vi "Main.vi"   [LabVIEW 2018]
doc: "Main interface to Dataflow DJ.\n\n<b>Execution System:</b> User Interface"
uses:
  Libraries/Audio Engine/Audio Engine.lvlib
  Libraries/Audio Output/Audio Output Queue Type.ctl
  Libraries/Audio Output/Audio Output.lvlib
  Libraries/Globals/Constants.vi
  Libraries/Globals/Globals.lvlib
  Libraries/User Interface/Sub Panels Cluster.ctl
  Libraries/User Interface/User Interface.lvlib
  Libraries/Config File/Config File.lvlib
  Libraries/Track Info/Track Info.lvlib
  Libraries/Track Info/Track Info FGV Enum.ctl
  Libraries/Track Info/Track Info.ctl
  Libraries/Config File/Config Cluster.ctl
  Plugins/Controllers/DAQmx/DAQmx.lvlib
  <vilib>/Analysis/NI_AALBase.lvlib
  <vilib>/Analysis/1siggen.llb/Ramp Pattern by Samples.vi
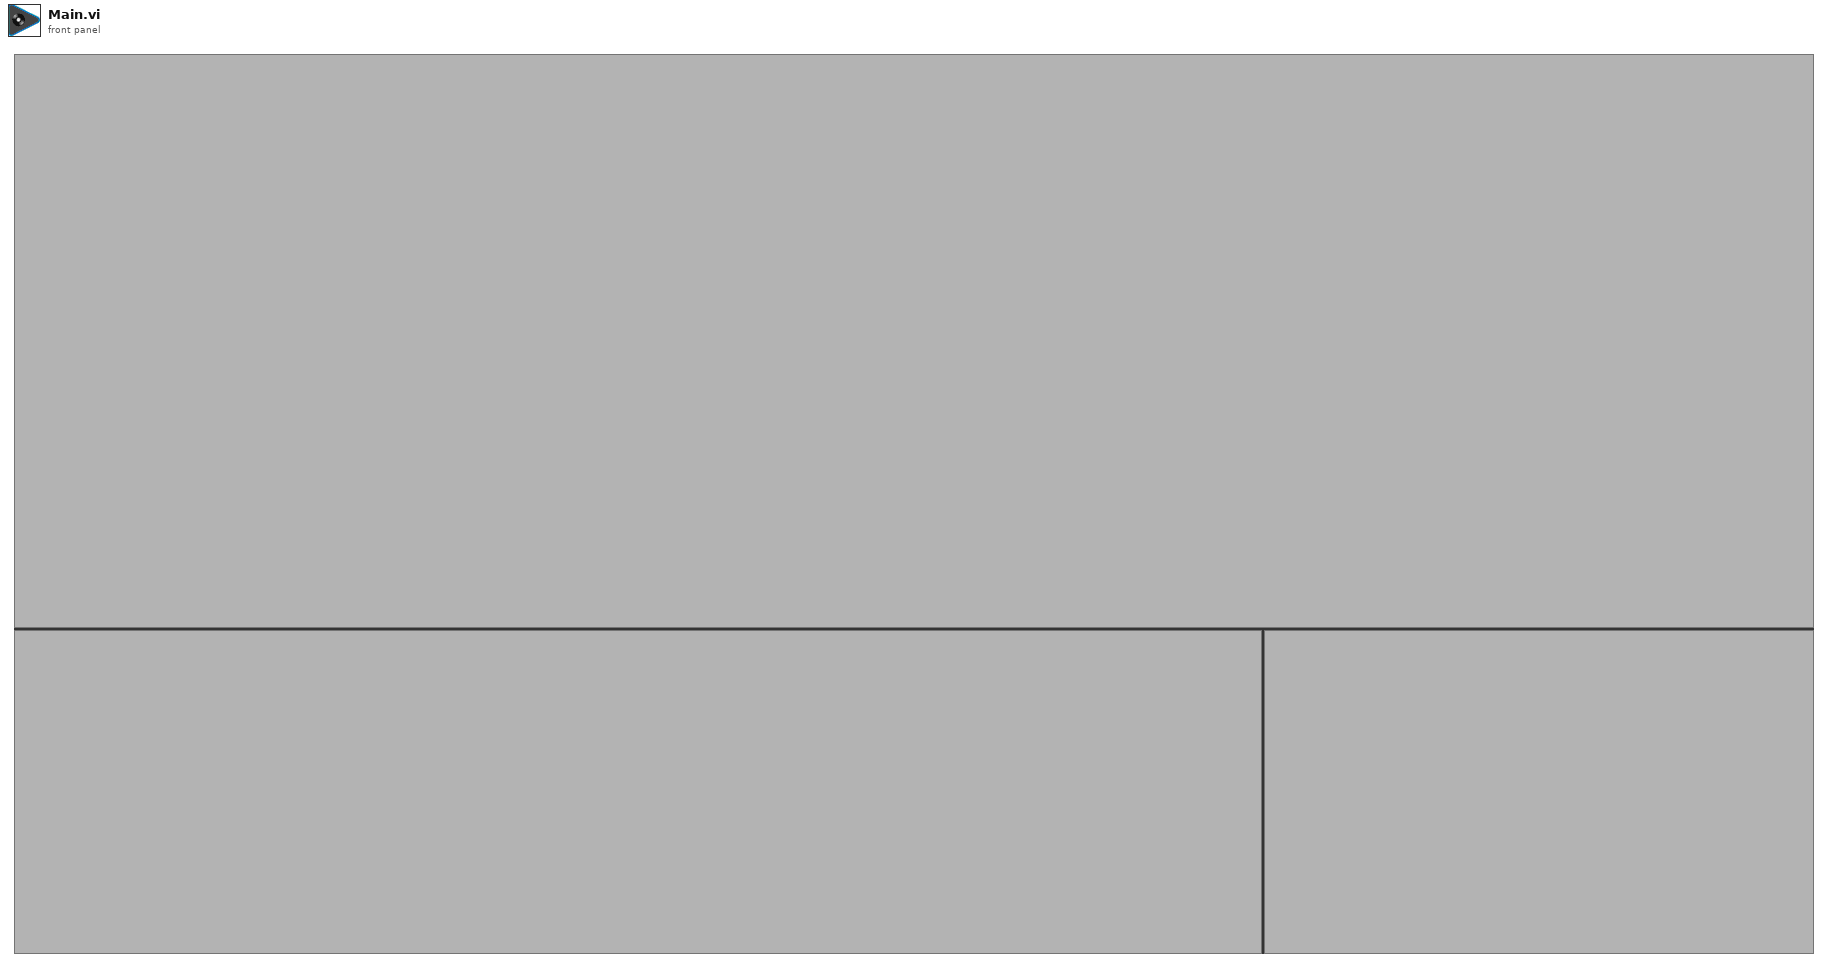
[diagram p1: front panel]
types:
  T1 = typedef "User Interface.lvlib/Sub Panels Cluster.ctl" = cluster{"DJ Interface":refnum<vi>, "File Browser":refnum<vi>, "Audio Config":refnum<vi>}
  T2 = typedef "Track Info.lvlib/Track Info FGV Enum.ctl" = enum16{"Init", "Update Track", "Update Multiple Tracks", "Get Track", "Get Multiple Tracks"}
  T3 = typedef "Audio Output.lvlib/Audio Output Queue Type.ctl" = cluster{"Master":waveform(i16)[], "Headphones":waveform(i16)[]}
  T4 = typedef "Config File.lvlib/Config Cluster.ctl" = cluster{"Track Info":T5[]}
  T5 = typedef "Track Info.lvlib/Track Info.ctl" = cluster{"Path":path, "Length (Samples)":i32, "Channels":i32, "Sample Rate (Hz)":i32, "BPM":dbl, "Cue Points (Samples)":i32[]}
  T6 = enum32{"invalid app kind", "Development System", "Run Time System", "Student Edition", "Embedded LabVIEW", "Evaluation", "Custom"}
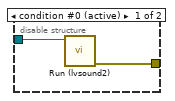
[diagram p4: hidden frame]
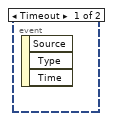
[diagram p5: hidden frame]
diagram:
  w10 = FALSE  # Shutdown
  # "Load WaveIO VIs programmatically\n\nif waveio.dll exists, then dynamically call VIs in waveio.llb\nif it doesn't exist, fall back to lvsound2.dll\n\nshould also address this issue"
  # "#TODO\nProgrammatically open reference to any VIs containing calls to DAQmx. Need to bundle those VIs with exe (block diagram included). Perform initial check for daqmx dll, and only then load VIs.\n\nUse PPLs to store code? Seem rather cumbersome to use. That said, if they're being loaded programmatically, they don't need to be linked in the project."
  # "Startup order required\nAudio Processing\n- Setup message queues for all control messages from UI and hardware\n- Begin generating output data\nAutio Output\n- Setup message queue from audio config UI panel\nUser Interface (DJ Interface)\n- Setup message queue to receive UI changes\n- Scan all UI elements and send values and limits to Audio Processing\nHardware Controller\n- Setup hardware and read current IO state\n- Send IO state to Audio Processing, which will then relay changes back to UI\n\n#TODO Use named Notifiers to wait for each component to start up"
  # "EXECUTION SYSTEMS\n\nAudio Processing.Run.vi    Standard\nAudio Output.Run.vi    Instrument I/O\nMain.vi    User Interface\nUser Interface.DJ Interface.vi    User Interface\nUser Interface.File Browser.vi    User Interface\nUser Interface.Audio Config.vi    User Interface\nHardware Control.DAQmx Run.vi    Data Acquisition\nAudio File Input.Load Async.vi    Other 1"
  # "Dataflow DJ - A live DJ mixing application written entirely in LabVIEW.\n    Copyright (C) 2019  Dataflow G\n    \n    This program is free software: you can redistribute it and/or modify\n    it under the terms of the GNU General Public License as published by\n    the Free Software Foundation, either version 3 of the License, or\n    (at your option) any later version.\n\n    This program is distributed in the hope that it will be useful,\n    but WITHOUT ANY WARRANTY; without even the implied warranty of\n    MERCHANTABILITY or FITNESS FOR A PARTICULAR PURPOSE.  See the\n    GNU General Public License for more details.\n\n    You should have received a copy of the GNU General Public License\n    along with this program.  If not, see <https://www.gnu.org/licenses/>.\n\nContact:\n    GitHub - https://github.com/dataflowg\n    Twitter - @Dataflow_G"
  # "If the WaveIO library is installed in external\\waveio_108, set WaveIO to TRUE in the Project's conditional disable symbols to use it here. \n\n#TODO\nAutomatically discover if WaveIO is available for development, maybe with a script or something."
  # "This is the main audio queue between the audio processing loop and audio output loop. It's a single element queue (SEQ) which contains the next block of audio data to be sent to both the master and headphone outputs. The block size is always Buffer Size (see global constant). Using a SEQ means the audio processing loop timing can be slaved to the audio output loop timing."
  # "Down, down, down. Would the fall NEVER come to an end!"
  n1 = flat-sequence {
    tunnel: [w27] -> w2
    frame #0 {
      # "Initialise Zero Buffer. This is sent to the soundcard when a track isn't loaded, is paused, or the headphone cue is disabled."
      n2 = global read "Constants.vi" "Buffer Size"() -> (w15:i32)
      n3 = global read "Constants.vi" "Channels"() -> (w16:i32)
      n4 = call "Track Info FGV.vi"("Track Info FGV Enum"=Track_Info_FGV_Enum."Init") -> ("error out"=w21:errorcluster)  [unwired: 7 in, 3 out]
      n5 = call-poly <vilib>:"Ramp Pattern.vi"("start"=0.0, "end"=1.0, "samples"=w15) -> ("Ramp Pattern"=w14:dbl[])  [unwired: 7 in, 1 out]
      n6 = call "Load Config.vi"("error in (no error)"=w21) -> ("Config"=w19:T4)  [unwired: 9 in, 1 out]
      n7 = Initialize Array(0.0, w16, w15) -> (w25:dbl[][])
      n8 = Unbundle By Name(w19) -> ("Track Info"=w23:T5[])
      n9 = Reverse 1D Array(array=w14) -> (reversed array=w13:dbl[])
      n10 = global write "Constants.vi" "Zero Buffer"(w25) -> ()
      n11 = global write "Constants.vi" "Ramp (Fade In)"(w14) -> ()
      n12 = global write "Constants.vi" "Ramp (Fade Out)"(w13) -> ()
      n13 = call "Track Info FGV.vi"("Track Info FGV Enum"=Track_Info_FGV_Enum."Update Multiple Tracks", "Multiple Track Info In"=w23) -> ()  [unwired: 6 in, 4 out]
    }
    frame #1 {
      n14 = Obtain Queue(max queue size (-1, unlimited)=1, name (unnamed)="Audio", element data type=T3 {"Master"=[], "Headphones"=[]}) -> (queue out=w27:refnum<queue>)  [unwired: 2 in, 2 out]
    }
  }
  n15 = control-ref of="DJ Interface Sub Panel"() -> (w8:refnum<vi>)
  n16 = control-ref of="File Browser Sub Panel"() -> (w7:refnum<vi>)
  n17 = control-ref of="Audio Config Sub Panel"() -> (w6:refnum<vi>)
  n18 = Bundle By Name(cluster=T1 {"DJ Interface"=refnum, "File Browser"=refnum, "Audio Config"=refnum} ("Sub Panels"), "DJ Interface"=w8, "File Browser"=w7, "Audio Config"=w6) -> (w5:T1)
  n19 = control-ref of="This VI"() -> (w4:refnum<vi>)
  n20 = Create User Event(user event datatype=w10) -> (user event=w1:refnum<user-event>, error out=w3:errorcluster)  [unwired: 1 in]
  n21 = call "Insert Sub Panels.vi"("error in (no error)"=w3, "Shutdown Event"=w1, "Sub Panels"=w5, "Owning VI"=w4) -> ()  [unwired: 7 in, 1 out]
  n22 = disable-structure shown="Disabled" {
    disable-tunnel: w1 -> [w31 _]
    frame Disabled {
      n23 = call "Check DAQmx Installed.vi"() -> ("DAQmx Installed?"=w30:bool)  [unwired: 10 in, 1 out]
      n24 = case shown="True" w30 {
        tunnel: w31 -> [_ w32]
        frame False {
        }
        frame True {
          n25 = call "Run.vi"("Shuwdown Event"=w32) -> ()  [unwired: 11 in]
        }
      }
    }
    frame Enabled {
    }
  }
  n26 = while {
    tunnel: w1 -> [w34]
    tunnel: w2 -> [w33]
    stop <- w35 stop-if-true
    n27 = event shown="[1] Panel Close?" {
      selector: _ -> [_ _]
      dyn-events: _ -> [_ _]
      timeout: _ -> [_ _]
      tunnel: [_ TRUE] -> w35
      tunnel: w34 -> [_ w47]
      tunnel: w33 -> [_ w41]
      event Timeout {
        n28 = event-data() -> ()  [unwired: 1 in, 3 out]
      }
      event Panel Close? {
        # "Write track info and config to disk on shutdown"
        # "Only close the panel if running under the run-time engine."
        n29 = event-data() -> ()  [unwired: 1 in, 4 out]
        n30 = Generate User Event(user event=w47, event data cluster=TRUE ("event data")) -> (user event out=w45:refnum<user-event>, error out=w44:errorcluster)  [unwired: 2 in]
        n31 = call "Track Info FGV.vi"("Track Info FGV Enum"=Track_Info_FGV_Enum."Get Multiple Tracks") -> ("Multiple Track Info Out"=w39:T5[])  [unwired: 7 in, 3 out]
        n32 = Destroy User Event(user event=w45, error in=w44) -> (error out=w40:errorcluster)
        n33 = Bundle By Name(cluster=T4 {"Track Info"=[]} ("Config"), "Track Info"=w39) -> (w38:T4)
        n34 = call "Save Config.vi"("Config"=w38) -> ()  [unwired: 10 in, 1 out]
        n35 = Release Queue(queue=w41, force destroy? (F)=TRUE, error in (no error)=w40) -> ()  [unwired: 3 out]
        n36 = property class="App"() -> ("App.Kind"=w50:T6)  [unwired: 2 in, 2 out]
        n37 = Not Equal?(x=w50, y=T6."Run Time System") -> (x != y?=w43:bool)
        n38 = event-data("Discard?"=w43) -> ()  [unwired: 1 in, 1 out]
      }
    }
  }
  n39 = disable-structure shown="WAVEIO==TRUE" {
    disable-tunnel: w2 -> [w52 w54]
    disable-tunnel: [w51 w53] -> w12
    frame condition #0 (active) {
      n40 = call "Run (lvsound2).vi"("Audio Output Queue"=w52) -> ("error out"=w51:errorcluster)  [unwired: 10 in]
    }
    frame condition #1 {
      n41 = call "Run (WaveIO).vi"("Audio Output Queue"=w54) -> ("error out"=w53:errorcluster)  [unwired: 10 in]
    }
  }
  n42 = call "Run.vi"("Audio Output Queue"=w2) -> ()  [unwired: 10 in, 1 out]
  n43 = call <vilib>:"General Error Handler.vi"("error in (no error)"=w12) -> ("error out"=w11:errorcluster)  [unwired: 10 in, 4 out]
  n44 = call ".vi"("error in (no escape)"=w11) -> ()
